vi "mxwScript_API_Option_SetStartDiagram(Path).vi"(8 "error in (no error)":errorcluster, 10 "path":string, 11 "options in":T1[](array[typedef])) -> (0 "error out":errorcluster, 3 "options out":T1[](array[typedef]))   [LabVIEW 2020]
doc: "Sets the password so password protected VIs can be generated into."
uses:
  codeGenAPISupport.llb/cgAPI_mxwScript_OptionData.ctl
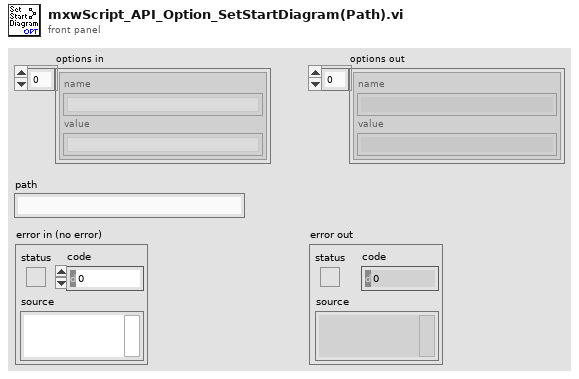
[diagram p1: front panel]
types:
  T1 = typedef "cgAPI_mxwScript_OptionData.ctl" = cluster{"name":string, "value":string}
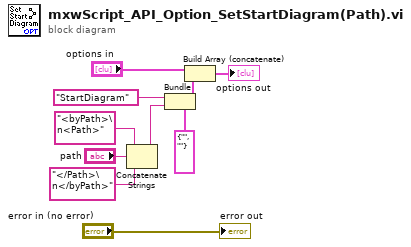
[diagram p0: block diagram]
diagram:
  n1 = Concatenate Strings("<byPath>\n<Path>", "path", "</Path>\n</byPath>") -> (w1:string)
  n2 = Bundle(cluster=T1 {"name"="", "value"=""} ("optionData"), "name"="StartDiagram", "value"=w1) -> (w8:T1)
  n3 = Build Array (concatenate)("options in", w8) -> (→"options out":T1[])
  "error out" <- "error in (no error)"
